vi "SC analysis.vi"(9 "Sampling Rate":dbl, 10 "Baseline":dbl, 11 "SC from sensor":dbl[](array[numeric])) -> (3 "Waveform Chart":dbl[](graph))   [LabVIEW 2014]
uses:
  <vilib>/addons/System Identification/Data Preprocess.llb/SI Lowpass Filter (SISO Array).vi
  <vilib>/addons/System Identification/NI_SysID.lvlib
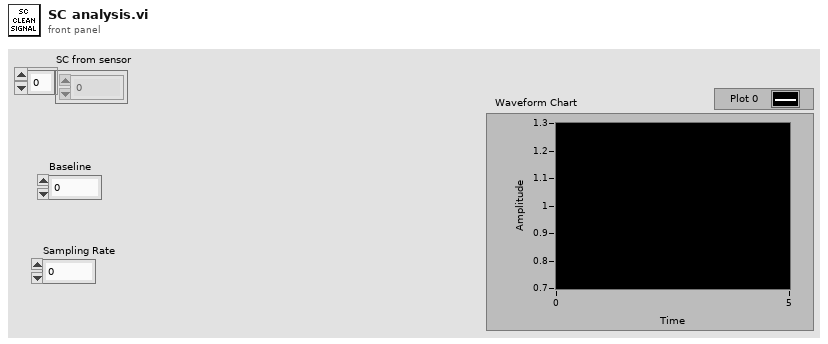
[diagram p1: front panel]
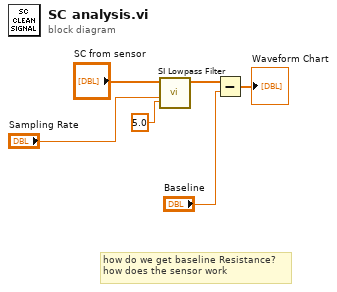
[diagram p0: block diagram]
diagram:
  # "how do we get baseline Resistance?\nhow does the sensor work"
  n1 = call-poly <vilib>:"SI Lowpass Filter.vi"("cutoff frequency"=5.0, "sampling rate (Hz)"="Sampling Rate", "stimulus signal in"="SC from sensor") -> ("stimulus signal out"=w4:dbl[])  [unwired: 6 in, 2 out]
  n2 = Subtract(x=w4, y="Baseline") -> (x-y=→"Waveform Chart":dbl[])
